vi "CloseFile.vi"(8 "error in (no error)":errorcluster, 9 "Action":enum16{"Prompt", "Keep", "Archive", "Trash"}(ring), 11 "Refnum in":refnum<k34>) -> (3 "File Close action out":enum16{"Prompt", "Keep", "Archive", "Trash"}(ring))   [LabVIEW 2018]
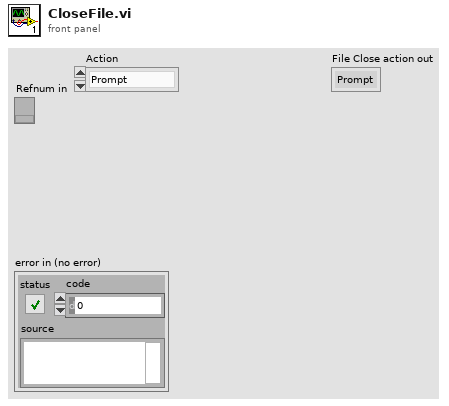
[diagram p1: front panel]
types:
  T1 = enum16{"Left Button", "Center Button", "Right Button", "Window Close"}
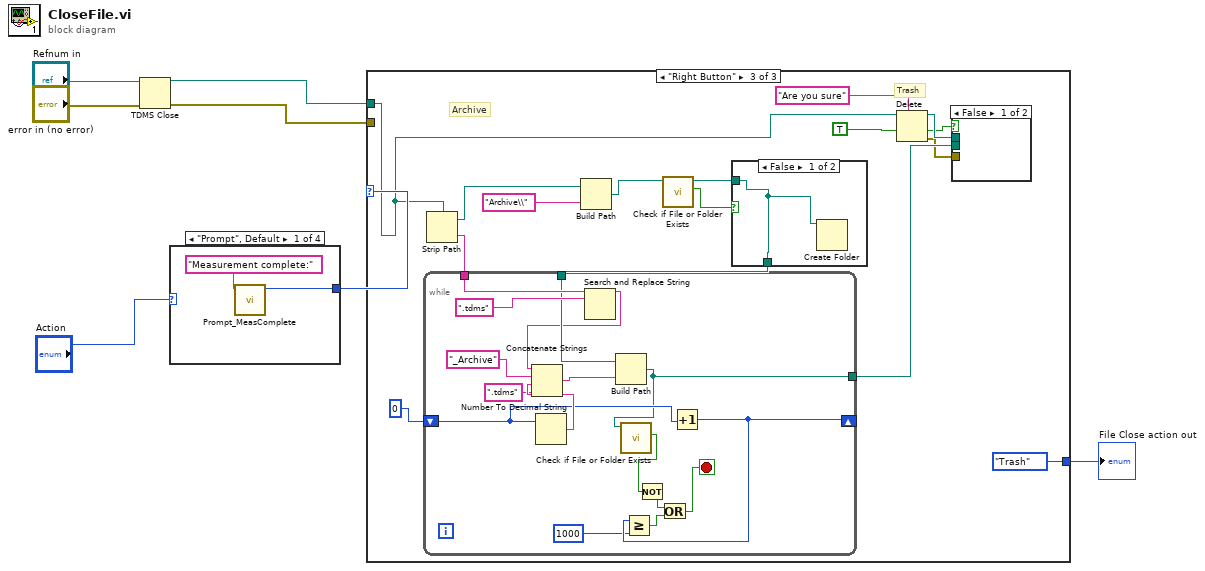
[diagram p0: block diagram]
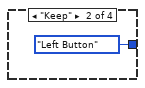
[diagram p2: hidden frame]
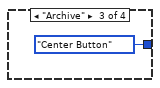
[diagram p3: hidden frame]
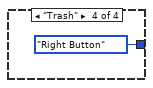
[diagram p4: hidden frame]
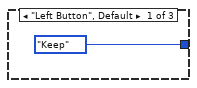
[diagram p5: hidden frame]
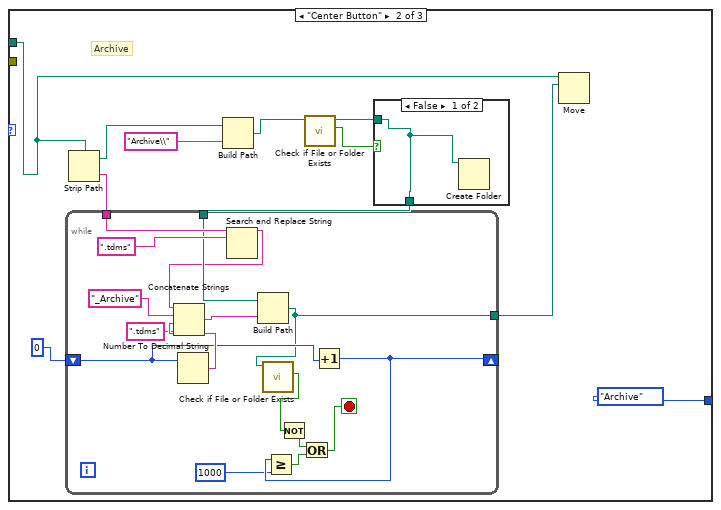
[diagram p6: hidden frame]
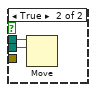
[diagram p8: hidden frame]
diagram:
  n1 = TDMS Close(8:"error in (no error)", 11:"Refnum in") -> (0:w7:errorcluster, 3:w6:path)
  n2 = case shown="\"Prompt\", Default" "Action" {
    tunnel: [w9 T1."Left Button" ("Which Button?") T1."Center Button" ("Which Button?") T1."Right Button" ("Which Button?")] -> w4
    frame "Prompt", Default {
      n3 = call "Prompt_MeasComplete.vi"("message"="Measurement complete:") -> ("Which Button?"=w9:T1)  [unwired: 10 in]
    }
    frame "Keep" {
    }
    frame "Archive" {
    }
    frame "Trash" {
    }
  }
  n4 = case shown="\"Right Button\"" w4 {
    tunnel: w6 -> [_ w14 w46]
    tunnel: w7 -> [_ _ _]
    tunnel: [enum16{"Prompt", "Keep", "Archive", "Trash"}."Keep" ("File Close action out") enum16{"Prompt", "Keep", "Archive", "Trash"}."Archive" ("File Close action out") enum16{"Prompt", "Keep", "Archive", "Trash"}."Trash" ("File Close action out")] -> w1
    frame "Left Button", Default {
    }
    frame "Center Button" {
      # "Archive"
      n5 = Strip Path(path=w14) -> (stripped path=w24:path, name=w22:string)
      n6 = Build Path(base path=w24, name or relative path="Archive\\") -> (appended path=w19:path)
      n7 = call <vilib>:"Check if File or Folder Exists.vi"("path"=w19) -> ("file or folder exists?"=w18:bool, "dup path"=w17:path)  [unwired: 8 in, 1 out]
      n8 = case shown="False" w18 {
        tunnel: w17 -> [w25 w26]
        tunnel: [w25 w26] -> w16
        frame False {
          n9 = Create Folder(path (use dialog)=w25) -> ()  [unwired: 2 in, 3 out]
        }
        frame True {
        }
      }
      n10 = while {
        tunnel: w22 -> [w42]
        tunnel: w16 -> [w40]
        shift-right: [w28] -> _
        shift-left: 0 -> [w34]
        tunnel: [w30] -> w20
        stop <- w31 stop-if-true
        n11 = Number To Decimal String(number=w34) -> (decimal integer string=w38:string)  [unwired: 1 in]
        n12 = Search and Replace String(input string=w42, search string=".tdms") -> (result string=w29:string)  [unwired: 6 in, 3 out]
        n13 = Concatenate Strings(w29, "_Archive" ("replace string (\"\")"), w38, ".tdms" ("string")) -> (w36:string)
        n14 = Build Path(base path=w40, name or relative path=w36) -> (appended path=w30:path)
        n15 = call <vilib>:"Check if File or Folder Exists.vi"("path"=w30) -> ("file or folder exists?"=w35:bool)  [unwired: 8 in, 2 out]
        n16 = Not(x=w35) -> (.not. x?=w33:bool)
        n17 = Increment(x=w34) -> (x+1=w28:i32)
        n18 = Greater Or Equal?(x=w28, y=1000) -> (x >= y?=w32:bool)
        n19 = Or(x=w33, y=w32) -> (x .or. y?=w31:bool)
      }
      n20 = Move(source path=w14, 10:w20) -> ()  [unwired: 3 in, 3 out]
    }
    frame "Right Button" {
      # "Trash"
      # "Archive"
      n21 = Strip Path(path=w46) -> (stripped path=w58:path, name=w56:string)
      n22 = Build Path(base path=w58, name or relative path="Archive\\") -> (appended path=w53:path)
      n23 = call <vilib>:"Check if File or Folder Exists.vi"("path"=w53) -> ("file or folder exists?"=w52:bool, "dup path"=w51:path)  [unwired: 8 in, 1 out]
      n24 = case shown="False" w52 {
        tunnel: w51 -> [w61 w62]
        tunnel: [w61 w62] -> w50
        frame False {
          n25 = Create Folder(path (use dialog)=w61) -> ()  [unwired: 2 in, 3 out]
        }
        frame True {
        }
      }
      n26 = while {
        tunnel: w56 -> [w78]
        tunnel: w50 -> [w76]
        shift-right: [w64] -> _
        shift-left: 0 -> [w70]
        tunnel: [w66] -> w54
        stop <- w67 stop-if-true
        n27 = Number To Decimal String(number=w70) -> (decimal integer string=w74:string)  [unwired: 1 in]
        n28 = Search and Replace String(input string=w78, search string=".tdms") -> (result string=w65:string)  [unwired: 6 in, 3 out]
        n29 = Concatenate Strings(w65, "_Archive" ("replace string (\"\")"), w74, ".tdms" ("string")) -> (w72:string)
        n30 = Build Path(base path=w76, name or relative path=w72) -> (appended path=w66:path)
        n31 = call <vilib>:"Check if File or Folder Exists.vi"("path"=w66) -> ("file or folder exists?"=w71:bool)  [unwired: 8 in, 2 out]
        n32 = Not(x=w71) -> (.not. x?=w69:bool)
        n33 = Increment(x=w70) -> (x+1=w64:i32)
        n34 = Greater Or Equal?(x=w64, y=1000) -> (x >= y?=w68:bool)
        n35 = Or(x=w69, y=w68) -> (x .or. y?=w67:bool)
      }
      n36 = Delete(prompt (Delete)="Are you sure", path (use dialog)=w46, confirm (F)=TRUE) -> (deleted path=w45:path, cancelled=w44:bool, error out=w43:errorcluster)  [unwired: 2 in]
      n37 = case shown="False" w44 {
        tunnel: w54 -> [_ w60]
        tunnel: w45 -> [_ w59]
        tunnel: w43 -> [_ _]
        frame False {
        }
        frame True {
          n38 = Move(source path=w59, 10:w60) -> ()  [unwired: 3 in, 3 out]
        }
      }
    }
  }
  "File Close action out" <- w1
